vi "template - FGV.vi"(8 "error in":errorcluster) -> (0 "error out":errorcluster)   [LabVIEW 2018]
doc: "Sends a message to all modules to abort and run shutdown code (with cleanup)."
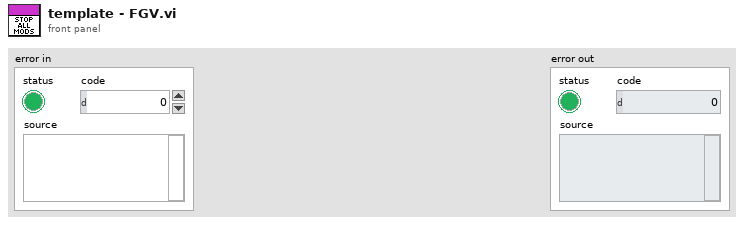
[diagram p1: front panel]
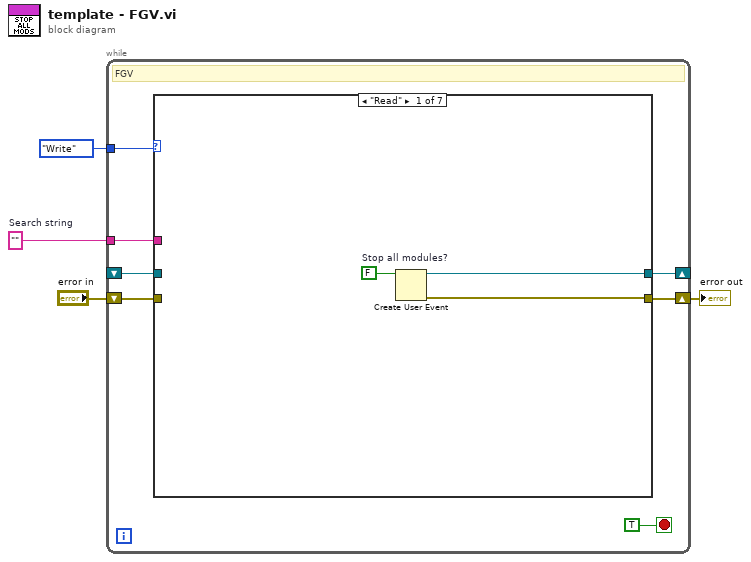
[diagram p0: block diagram]
diagram:
  w1 = ""  # Search string
  n1 = while {
    tunnel: enum16{"Read", "Search", "Write"}."Write" -> [w11]
    shift-right: [w9] -> _
    shift-left: _ -> [w8]
    shift-right: [w7] -> w2
    shift-left: "error in" -> [w6]
    tunnel: w1 -> [w5]
    stop <- TRUE stop-if-true
    # "FGV"
    n2 = case shown="\"Create\"" w11 {
      tunnel: [w13 _ _ _ _ _ _] -> w9
      tunnel: w8 -> [_ _ _ _ _ _ _]
      tunnel: [w12 _ _ _ _ _ _] -> w7
      tunnel: w6 -> [_ _ _ _ _ _ _]
      tunnel: w5 -> [_ _ _ _ _ _ _]
      frame "Read" {
        w14 = FALSE  # Stop all modules?
        n3 = Create User Event(user event datatype=w14) -> (user event=w13:refnum<user-event>, error out=w12:errorcluster)  [unwired: 1 in]
      }
      frame "Search" {
      }
      frame "Search" {
      }
      frame "Write", Default {
      }
      frame "Read" {
      }
      frame "Search" {
      }
      frame "Write" {
      }
    }
  }
  "error out" <- w2
